vi "Device Managing.vi"() -> ()   [LabVIEW 2022 SP3]
uses:
  VideoCard.ctl
  ScanningControl/Motion Controllers/-MotionRoutines/MotionGlobals.vi
  <vilib>/regexp/Match Regular Expression.xnode
panel:
  out "error out 2":errorcluster
  out "NVIDIA Card":T1
  out "standard output":string
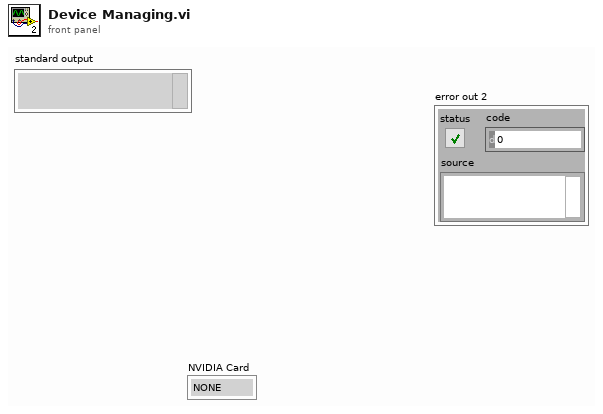
[diagram p1: front panel]
types:
  T1 = typedef "VideoCard.ctl" = enum16{"NONE", "UNKNOWN", "k620", "FX 3800", "GTX 970", "P1000"}
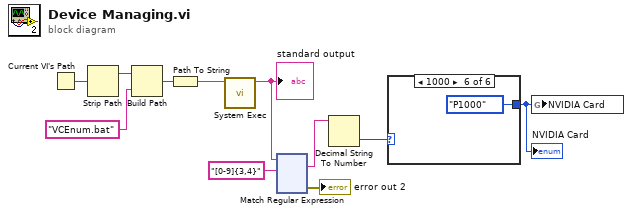
[diagram p0: block diagram]
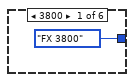
[diagram p2: hidden frame]
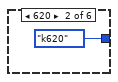
[diagram p3: hidden frame]
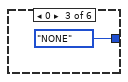
[diagram p4: hidden frame]
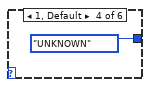
[diagram p5: hidden frame]
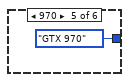
[diagram p6: hidden frame]
diagram:
  n1 = Current VI's Path() -> (path=w11:path)
  n2 = Strip Path(path=w11) -> (stripped path=w10:path)  [unwired: 1 out]
  n3 = Build Path(base path=w10, name or relative path="VCEnum.bat") -> (appended path=w8:path)
  n4 = Path To String(path=w8) -> (string=w7:string)
  n5 = call <vilib>:"System Exec.vi"("command line"=w7) -> ("standard output"=w6:string)  [unwired: 7 in, 3 out]
  "standard output" <- w6
  n6 = xnode "Match Regular Expression"("input string"=w6, "regular expression"="[0-9]{3,4}") -> ("whole match"=w2:string, "error out"=→"error out 2":errorcluster)  [unwired: 4 in, 3 out]
  n7 = Decimal String To Number(string=w2) -> (number=w3:i32)  [unwired: 2 in, 1 out]
  n8 = case shown="1000" w3 {
    tunnel: [VideoCard."FX 3800" ("NVIDIA Card") VideoCard."k620" ("NVIDIA Card") VideoCard."NONE" ("NVIDIA Card") VideoCard."UNKNOWN" ("NVIDIA Card") VideoCard."GTX 970" ("NVIDIA Card") VideoCard."P1000" ("NVIDIA Card")] -> w1
    frame 3800 {
    }
    frame 620 {
    }
    frame 0 {
    }
    frame 1, Default {
    }
    frame 970 {
    }
    frame 1000 {
    }
  }
  "NVIDIA Card" <- w1
  n9 = global write "MotionGlobals.vi" "NVIDIA Card"(w1) -> ()
